vi "PC-Beamage Labview Example.vi"() -> ()   [LabVIEW 2013]
panel:
  in  "Manual":bool
  in  "Auto":bool
  in  "save current image":bool caption="Capture"
  in  "subtract background":bool caption="Capture"
  in  "ms":dbl=200.0 min=0.06 max=200.0 step=0.01
  in  "1ovre on":bool
  in  "FWHM On":bool
  in  "Log on":bool
  in  "Gauss on":bool
  in  "1ovre":bool
  in  "FWHM":bool
  in  "Log":bool
  in  "Gauss":bool caption="Press to Activate Measurements"
  in  "Display":T1(ring) caption="Press Buttons to Activate XY Measurements"
  in  "Time out":i32
  out "ok for com":bool
  out "DLL Present":bool
  out "Connected":bool
  in  "Common Measurements":T2(ring)
  out "Common Measurement":string caption="Effective Diameter"
  in  "Y Axis Measurements":T3(ring)
  in  "X Axis Measurements":T3(ring)
  out "Camera Serial Number":string
  out "PC Beamage Version":string caption="PC Beamage SW Version"
  out "Y Axis Measurement":string caption="Y Axis Centroid"
  out "X Axis Measurement":string caption="X Axis Centroid"
  in  "exit":bool
  in  "Orientation :":enum16{"Auto Orient", "0 Degrees", "45 Degress"}(ring)
  in  "Center :":enum16{"Centroid", "Peak"}(ring)
  in  "start capture":bool caption="Capture"
  in  "disconnect":bool
  in  "connect":bool
  in  "Definition :":T4(ring)
  # "PC-Beamage Labview Control Example"
  # "Main Controls"
  # "Measures"
  # "Exposure Time"
  # "Select Measurements to Display"
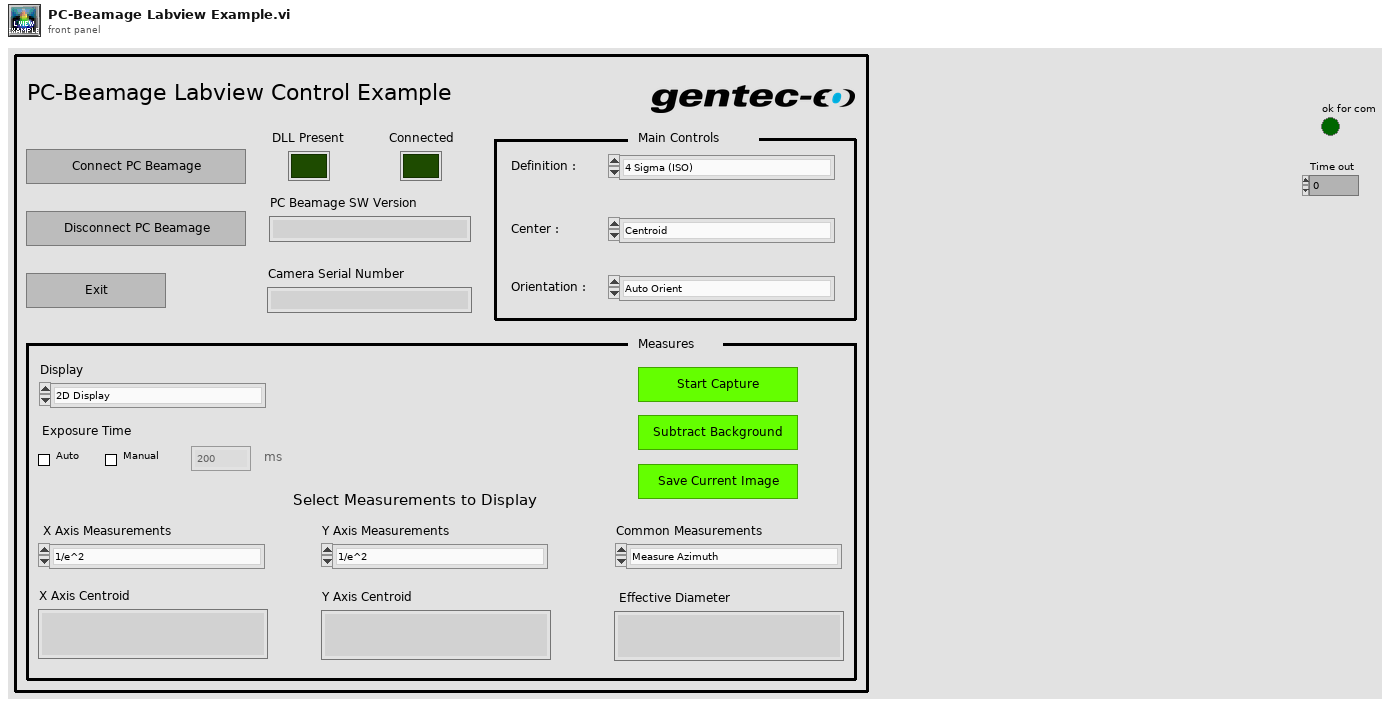
[diagram p1: front panel]
types:
  T1 = enum16{"2D Display", "3D Display", "XY Display", "Beam Track Display"}
  T2 = enum16{"Measure Azimuth", "Measure Delta", "Measure Effective Diameter", "Measure Ellipticity", "Measure Number of Samples", "Measure Orientation", "Measure Peak Saturation", "Measure Minor Axis", "Measure Major Axis", "Measure RMS", ""}
  T3 = enum16{"1/e^2", "Centroid", "Delta", "FWHM", "Gaussian Equation", "Gaussian % Fit", "Roughness Fit", "Last", "Mean", "Peak to Average Ratio", "Peak"}
  T4 = enum16{"4 Sigma (ISO)", "FWHM along Crosshairs (50%)", "1 / e^2 along Crosshairs (13.5%)", "86 % effective Diameter"}
  T5 = enum8{"Enabled", "Disabled", "Disabled and Grayed Out"}
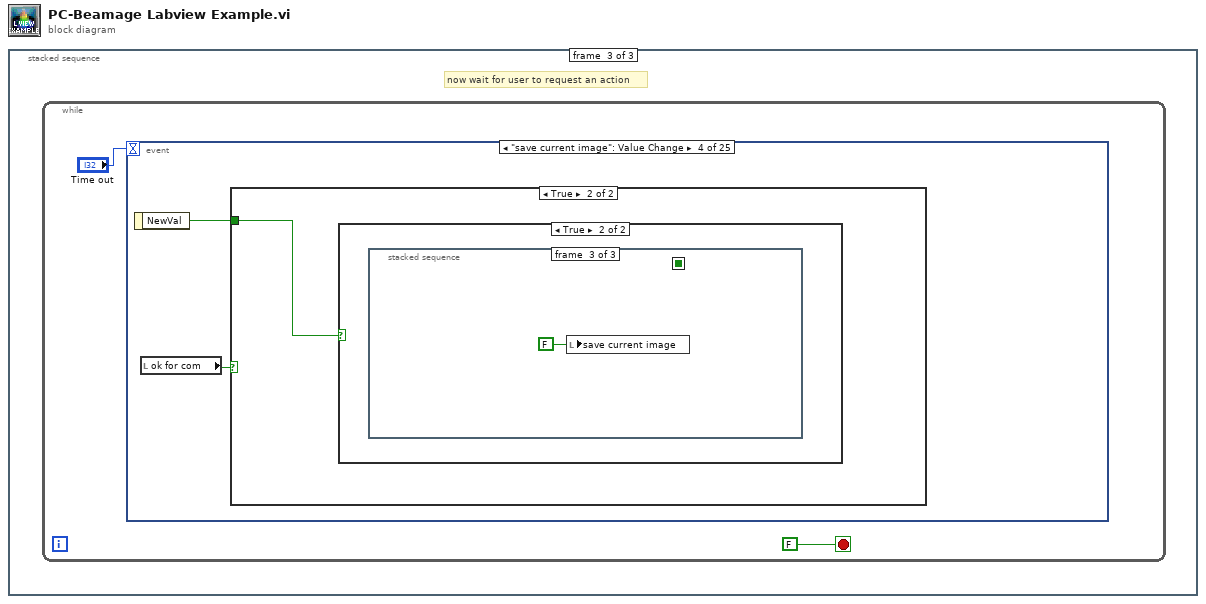
[diagram p0: block diagram]
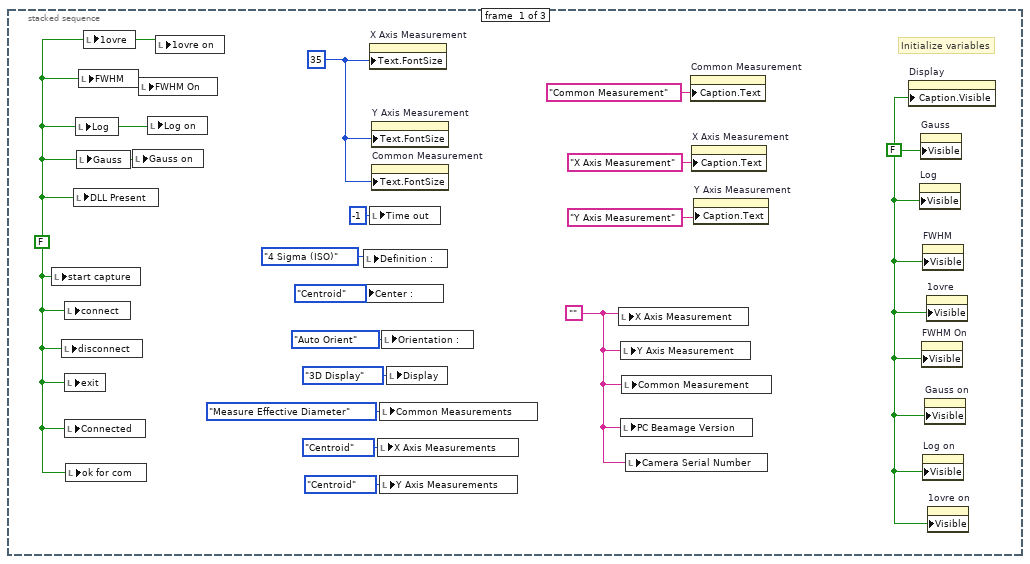
[diagram p2: hidden frame]
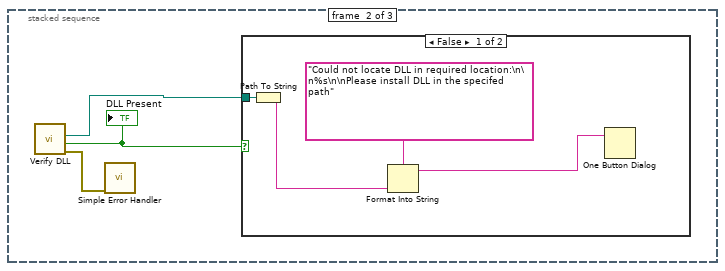
[diagram p3: hidden frame]
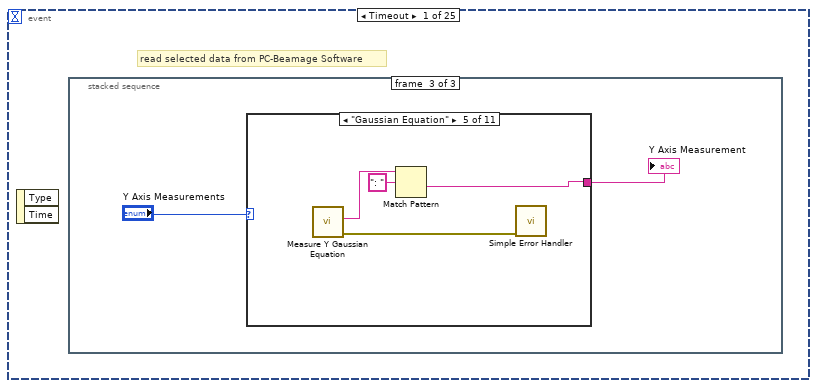
[diagram p5: hidden frame]
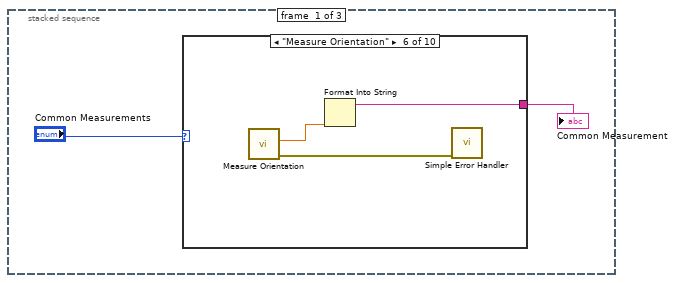
[diagram p6: hidden frame]
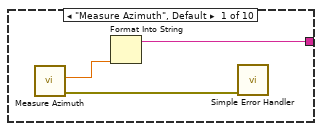
[diagram p7: hidden frame]
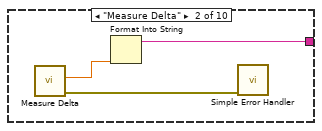
[diagram p8: hidden frame]
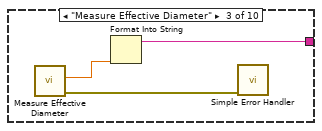
[diagram p9: hidden frame]
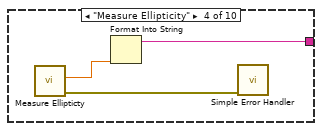
[diagram p10: hidden frame]
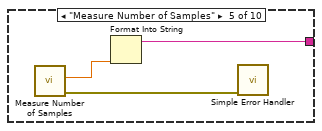
[diagram p11: hidden frame]
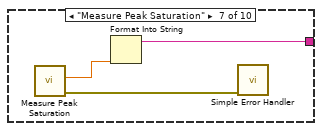
[diagram p12: hidden frame]
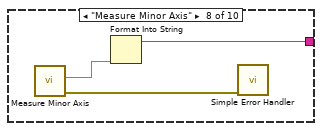
[diagram p13: hidden frame]
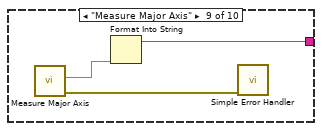
[diagram p14: hidden frame]
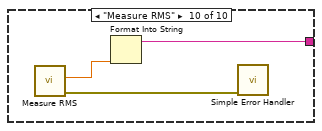
[diagram p15: hidden frame]
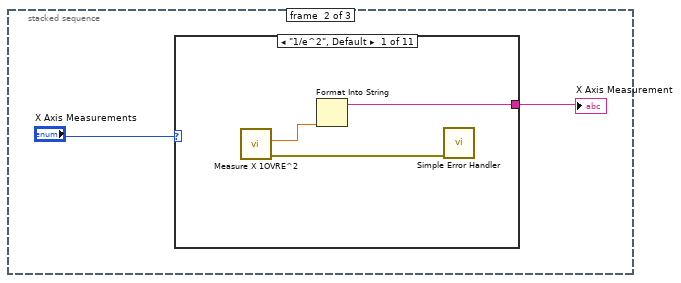
[diagram p16: hidden frame]
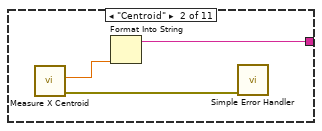
[diagram p17: hidden frame]
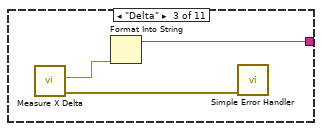
[diagram p18: hidden frame]
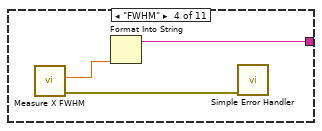
[diagram p19: hidden frame]
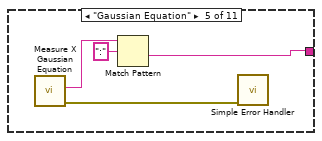
[diagram p20: hidden frame]
diagram:
  n1 = stacked-sequence {
    frame #0 {
      w3 = FALSE ("Visible")
      w7 = u32 35 ("Text.Font:Size")
      w4 = FALSE ("verifiy dll")
      w15 = ""
      # "Initialize variables"
      n2 = local write "start capture"(w4) -> ()
      n3 = local write "disconnect"(w4) -> ()
      n4 = local write "connect"(w4) -> ()
      n5 = local write "exit"(w4) -> ()
      n6 = local write "Connected"(w4) -> ()
      n7 = local write "ok for com"(w4) -> ()
      n8 = local write "DLL Present"(w4) -> ()
      n9 = local write "Log"(w4) -> ()
      n10 = local write "Gauss"(w4) -> ()
      n11 = local write "FWHM"(w4) -> ()
      n12 = local write "1ovre"(w4) -> ()
      n13 = local write "Gauss on"(w4) -> ()
      n14 = local write "FWHM On"(w4) -> ()
      n15 = local write "Log on"(w4) -> ()
      n16 = local write "1ovre on"(w4) -> ()
      n17 = local write "Center :"(enum16{"Centroid", "Peak"}."Centroid" ("Center :")) -> ()
      n18 = local write "Definition :"(T4."4 Sigma (ISO)" ("Definition :")) -> ()
      n19 = property on="X Axis Measurement" class="Str"("Text.FontSize"=w7) -> ()  [unwired: 2 in, 2 out]
      n20 = local write "Time out"(-1 ("Time out")) -> ()
      n21 = property on="Y Axis Measurement" class="Str"("Text.FontSize"=w7) -> ()  [unwired: 2 in, 2 out]
      n22 = property on="Common Measurement" class="Str"("Text.FontSize"=w7) -> ()  [unwired: 2 in, 2 out]
      n23 = local write "X Axis Measurements"(T3."Centroid" ("X Axis Measurements")) -> ()
      n24 = local write "Common Measurements"(T2."Measure Effective Diameter" ("Common Measurements")) -> ()
      n25 = local write "Y Axis Measurements"(T3."Centroid" ("Y Axis Measurements")) -> ()
      n26 = local write "Orientation :"(enum16{"Auto Orient", "0 Degrees", "45 Degress"}."Auto Orient" ("Orientation :")) -> ()
      n27 = local write "Display"(T1."3D Display" ("Display")) -> ()
      n28 = local write "X Axis Measurement"(w15) -> ()
      n29 = local write "Y Axis Measurement"(w15) -> ()
      n30 = local write "PC Beamage Version"(w15) -> ()
      n31 = local write "Common Measurement"(w15) -> ()
      n32 = local write "Camera Serial Number"(w15) -> ()
      n33 = property on="Common Measurement" class="Str"("Caption.Text"="Common Measurement") -> ()  [unwired: 2 in, 2 out]
      n34 = property on="X Axis Measurement" class="Str"("Caption.Text"="X Axis Measurement") -> ()  [unwired: 2 in, 2 out]
      n35 = property on="Y Axis Measurement" class="Str"("Caption.Text"="Y Axis Measurement") -> ()  [unwired: 2 in, 2 out]
      n36 = property on="Display" class="Enum (strict)"("Caption.Visible"=w3) -> ()  [unwired: 2 in, 2 out]
      n37 = property on="Log" class="Bool (strict)"("Visible"=w3) -> ()  [unwired: 2 in, 2 out]
      n38 = property on="Gauss" class="Bool (strict)"("Visible"=w3) -> ()  [unwired: 2 in, 2 out]
      n39 = property on="FWHM On" class="Bool (strict)"("Visible"=w3) -> ()  [unwired: 2 in, 2 out]
      n40 = property on="FWHM" class="Bool (strict)"("Visible"=w3) -> ()  [unwired: 2 in, 2 out]
      n41 = property on="Log on" class="Bool (strict)"("Visible"=w3) -> ()  [unwired: 2 in, 2 out]
      n42 = property on="Gauss on" class="Bool (strict)"("Visible"=w3) -> ()  [unwired: 2 in, 2 out]
      n43 = property on="1ovre" class="Bool (strict)"("Visible"=w3) -> ()  [unwired: 2 in, 2 out]
      n44 = property on="1ovre on" class="Bool (strict)"("Visible"=w3) -> ()  [unwired: 2 in, 2 out]
    }
    frame #1 {
      n45 = call "Verify DLL.vi"() -> ("error out"=w16:errorcluster, "DLL is Present"=w18:bool, "path"=w17:path)  [unwired: 9 in]
      "DLL Present" <- w18
      n46 = call <vilib>:"Simple Error Handler.vi"("error in (no error)"=w16) -> ()  [unwired: 4 in, 5 out]
      n47 = case shown="False" w18 {
        tunnel: w17 -> [w22 _]
        frame False {
          n48 = Path To String(path=w22) -> (string=w20:string)
          n49 = Format Into String(format string="Could not locate DLL in required location:\n\n%s\n\nPlease install DLL in the specifed path", w20) -> (resulting string=w19:string)  [unwired: 2 in, 1 out]
          n50 = One Button Dialog(message=w19) -> ()  [unwired: 1 in, 1 out]
        }
        frame True {
        }
      }
    }
    frame #2 {
      # "now wait for user to request an action"
      n51 = while {
        stop <- FALSE stop-if-true
        n52 = event shown="[3] \"save current image\": Value Change" {
          selector: _ -> [_ _ _ _ _ _ _ _ _ _ _ _ _ _ _ _ _ _ _ _ _ _ _ _ _]
          dyn-events: _ -> [_ _ _ _ _ _ _ _ _ _ _ _ _ _ _ _ _ _ _ _ _ _ _ _ _]
          timeout: "Time out" -> [_ _ _ _ _ _ _ _ _ _ _ _ _ _ _ _ _ _ _ _ _ _ _ _ _]
          event Timeout {
            # "read selected data from PC-Beamage Software"
            n53 = event-data() -> ()  [unwired: 1 in, 2 out]
            n54 = stacked-sequence {
              frame #0 {
                n55 = case shown="\"Measure Orientation\"" "Common Measurements" {
                  tunnel: [w27 w30 w33 w36 w39 w42 w45 w48 w51 w54] -> w25
                  frame "Measure Azimuth", Default {
                    n56 = call "Measure Azimuth.vi"() -> ("error out"=w29:errorcluster, "Azimuth"=w28:dbl)  [unwired: 10 in]
                    n57 = Format Into String(w28) -> (resulting string=w27:string)  [unwired: 3 in, 1 out]
                    n58 = call <vilib>:"Simple Error Handler.vi"("error in (no error)"=w29) -> ()  [unwired: 4 in, 5 out]
                  }
                  frame "Measure Delta" {
                    n59 = call "Measure Delta.vi"() -> ("error out"=w32:errorcluster, "Delta"=w31:dbl)  [unwired: 10 in]
                    n60 = Format Into String(w31) -> (resulting string=w30:string)  [unwired: 3 in, 1 out]
                    n61 = call <vilib>:"Simple Error Handler.vi"("error in (no error)"=w32) -> ()  [unwired: 4 in, 5 out]
                  }
                  frame "Measure Effective Diameter" {
                    n62 = call "Measure Effective Diameter.vi"() -> ("error out"=w35:errorcluster, "Effective Diameter"=w34:dbl)  [unwired: 10 in]
                    n63 = Format Into String(w34) -> (resulting string=w33:string)  [unwired: 3 in, 1 out]
                    n64 = call <vilib>:"Simple Error Handler.vi"("error in (no error)"=w35) -> ()  [unwired: 4 in, 5 out]
                  }
                  frame "Measure Ellipticity" {
                    n65 = call "Measure Ellipticty.vi"() -> ("error out"=w38:errorcluster, "Ellipticity"=w37:dbl)  [unwired: 10 in]
                    n66 = Format Into String(w37) -> (resulting string=w36:string)  [unwired: 3 in, 1 out]
                    n67 = call <vilib>:"Simple Error Handler.vi"("error in (no error)"=w38) -> ()  [unwired: 4 in, 5 out]
                  }
                  frame "Measure Number of Samples" {
                    n68 = call "Measure Number of Samples.vi"() -> ("error out"=w41:errorcluster, "Number of Samples"=w40:dbl)  [unwired: 10 in]
                    n69 = Format Into String(w40) -> (resulting string=w39:string)  [unwired: 3 in, 1 out]
                    n70 = call <vilib>:"Simple Error Handler.vi"("error in (no error)"=w41) -> ()  [unwired: 4 in, 5 out]
                  }
                  frame "Measure Orientation" {
                    n71 = call "Measure Orientation.vi"() -> ("error out"=w44:errorcluster, "Orienttion"=w43:dbl)  [unwired: 10 in]
                    n72 = Format Into String(w43) -> (resulting string=w42:string)  [unwired: 3 in, 1 out]
                    n73 = call <vilib>:"Simple Error Handler.vi"("error in (no error)"=w44) -> ()  [unwired: 4 in, 5 out]
                  }
                  frame "Measure Peak Saturation" {
                    n74 = call "Measure Peak Saturation.vi"() -> ("error out"=w47:errorcluster, "Peak Saturation"=w46:dbl)  [unwired: 10 in]
                    n75 = Format Into String(w46) -> (resulting string=w45:string)  [unwired: 3 in, 1 out]
                    n76 = call <vilib>:"Simple Error Handler.vi"("error in (no error)"=w47) -> ()  [unwired: 4 in, 5 out]
                  }
                  frame "Measure Minor Axis" {
                    n77 = call "Measure Minor Axis.vi"() -> ("error out"=w50:errorcluster, "Minor Axis"=w49:dbl)  [unwired: 10 in]
                    n78 = Format Into String(w49) -> (resulting string=w48:string)  [unwired: 3 in, 1 out]
                    n79 = call <vilib>:"Simple Error Handler.vi"("error in (no error)"=w50) -> ()  [unwired: 4 in, 5 out]
                  }
                  frame "Measure Major Axis" {
                    n80 = call "Measure Major Axis.vi"() -> ("error out"=w53:errorcluster, "Major Axis"=w52:dbl)  [unwired: 10 in]
                    n81 = Format Into String(w52) -> (resulting string=w51:string)  [unwired: 3 in, 1 out]
                    n82 = call <vilib>:"Simple Error Handler.vi"("error in (no error)"=w53) -> ()  [unwired: 4 in, 5 out]
                  }
                  frame "Measure RMS" {
                    n83 = call "Measure RMS.vi"() -> ("error out"=w56:errorcluster, "RMS"=w55:dbl)  [unwired: 10 in]
                    n84 = Format Into String(w55) -> (resulting string=w54:string)  [unwired: 3 in, 1 out]
                    n85 = call <vilib>:"Simple Error Handler.vi"("error in (no error)"=w56) -> ()  [unwired: 4 in, 5 out]
                  }
                }
                "Common Measurement" <- w25
              }
              frame #1 {
                n86 = case shown="\"1/e^2\", Default" "X Axis Measurements" {
                  tunnel: [w59 w62 w65 w68 w71 w75 w78 w81 w84 w87 w90] -> w58
                  frame "1/e^2", Default {
                    n87 = call "Measure X 1OVRE^2.vi"() -> ("error out"=w61:errorcluster, "X 1/E^2"=w60:dbl)  [unwired: 10 in]
                    n88 = Format Into String(w60) -> (resulting string=w59:string)  [unwired: 3 in, 1 out]
                    n89 = call <vilib>:"Simple Error Handler.vi"("error in (no error)"=w61) -> ()  [unwired: 4 in, 5 out]
                  }
                  frame "Centroid" {
                    n90 = call "Measure X Centroid.vi"() -> ("error out"=w64:errorcluster, "X Centroid"=w63:dbl)  [unwired: 10 in]
                    n91 = Format Into String(w63) -> (resulting string=w62:string)  [unwired: 3 in, 1 out]
                    n92 = call <vilib>:"Simple Error Handler.vi"("error in (no error)"=w64) -> ()  [unwired: 4 in, 5 out]
                  }
                  frame "Delta" {
                    n93 = call "Measure X Delta.vi"() -> ("error out"=w67:errorcluster, "X Delta"=w66:dbl)  [unwired: 10 in]
                    n94 = Format Into String(w66) -> (resulting string=w65:string)  [unwired: 3 in, 1 out]
                    n95 = call <vilib>:"Simple Error Handler.vi"("error in (no error)"=w67) -> ()  [unwired: 4 in, 5 out]
                  }
                  frame "FWHM" {
                    n96 = call "Measure X FWHM.vi"() -> ("error out"=w70:errorcluster, "X FWHM"=w69:dbl)  [unwired: 10 in]
                    n97 = Format Into String(w69) -> (resulting string=w68:string)  [unwired: 3 in, 1 out]
                    n98 = call <vilib>:"Simple Error Handler.vi"("error in (no error)"=w70) -> ()  [unwired: 4 in, 5 out]
                  }
                  frame "Gaussian Equation" {
                    n99 = call "Measure X Gaussian Equation.vi"() -> ("error out"=w74:errorcluster, "X Gaussian Equation"=w73:string)  [unwired: 10 in]
                    n100 = Match Pattern(string=w73, regular expression=":") -> (after substring=w71:string)  [unwired: 1 in, 3 out]
                    n101 = call <vilib>:"Simple Error Handler.vi"("error in (no error)"=w74) -> ()  [unwired: 4 in, 5 out]
                  }
                  frame "Gaussian % Fit" {
                    n102 = call "Measure X Gaussian Fit %.vi"() -> ("error out"=w77:errorcluster, "X Gaussian Fit %"=w76:dbl)  [unwired: 10 in]
                    n103 = Format Into String(w76) -> (resulting string=w75:string)  [unwired: 3 in, 1 out]
                    n104 = call <vilib>:"Simple Error Handler.vi"("error in (no error)"=w77) -> ()  [unwired: 4 in, 5 out]
                  }
                  frame "Roughness Fit" {
                    n105 = call "Measure X Roughness Fit.vi"() -> ("error out"=w80:errorcluster, "X Roughness Fit"=w79:dbl)  [unwired: 10 in]
                    n106 = Format Into String(w79) -> (resulting string=w78:string)  [unwired: 3 in, 1 out]
                    n107 = call <vilib>:"Simple Error Handler.vi"("error in (no error)"=w80) -> ()  [unwired: 4 in, 5 out]
                  }
                  frame "Last" {
                    n108 = call "Measure X Last.vi"() -> ("error out"=w83:errorcluster, "X Last"=w82:dbl)  [unwired: 10 in]
                    n109 = Format Into String(w82) -> (resulting string=w81:string)  [unwired: 3 in, 1 out]
                    n110 = call <vilib>:"Simple Error Handler.vi"("error in (no error)"=w83) -> ()  [unwired: 4 in, 5 out]
                  }
                  frame "Mean" {
                    n111 = call "Measure X Mean.vi"() -> ("error out"=w86:errorcluster, "X Mean"=w85:dbl)  [unwired: 10 in]
                    n112 = Format Into String(w85) -> (resulting string=w84:string)  [unwired: 3 in, 1 out]
                    n113 = call <vilib>:"Simple Error Handler.vi"("error in (no error)"=w86) -> ()  [unwired: 4 in, 5 out]
                  }
                  frame "Peak to Average Ratio" {
                    n114 = call "Measure X Peak to Average.vi"() -> ("error out"=w89:errorcluster, "X Peak to Average Ratio"=w88:dbl)  [unwired: 10 in]
                    n115 = Format Into String(w88) -> (resulting string=w87:string)  [unwired: 3 in, 1 out]
                    n116 = call <vilib>:"Simple Error Handler.vi"("error in (no error)"=w89) -> ()  [unwired: 4 in, 5 out]
                  }
                  frame "Peak" {
                    n117 = call "Measure X Peak.vi"() -> ("error out"=w92:errorcluster, "X Peak"=w91:dbl)  [unwired: 10 in]
                    n118 = Format Into String(w91) -> (resulting string=w90:string)  [unwired: 3 in, 1 out]
                    n119 = call <vilib>:"Simple Error Handler.vi"("error in (no error)"=w92) -> ()  [unwired: 4 in, 5 out]
                  }
                }
                "X Axis Measurement" <- w58
              }
              frame #2 {
                n120 = case shown="\"Gaussian Equation\"" "Y Axis Measurements" {
                  tunnel: [w95 w98 w101 w104 w107 w111 w114 w117 w120 w123 w126] -> w93
                  frame "1/e^2", Default {
                    n121 = call "Measure Y 1OVRE^2.vi"() -> ("error out"=w97:errorcluster, "Y 1/E^2"=w96:dbl)  [unwired: 10 in]
                    n122 = Format Into String(w96) -> (resulting string=w95:string)  [unwired: 3 in, 1 out]
                    n123 = call <vilib>:"Simple Error Handler.vi"("error in (no error)"=w97) -> ()  [unwired: 4 in, 5 out]
                  }
                  frame "Centroid" {
                    n124 = call "Measure Y Centroid.vi"() -> ("error out"=w100:errorcluster, "Y Centroid"=w99:dbl)  [unwired: 10 in]
                    n125 = Format Into String(w99) -> (resulting string=w98:string)  [unwired: 3 in, 1 out]
                    n126 = call <vilib>:"Simple Error Handler.vi"("error in (no error)"=w100) -> ()  [unwired: 4 in, 5 out]
                  }
                  frame "Delta" {
                    n127 = call "Measure Y Delta.vi"() -> ("error out"=w103:errorcluster, "Y Delta"=w102:dbl)  [unwired: 10 in]
                    n128 = Format Into String(w102) -> (resulting string=w101:string)  [unwired: 3 in, 1 out]
                    n129 = call <vilib>:"Simple Error Handler.vi"("error in (no error)"=w103) -> ()  [unwired: 4 in, 5 out]
                  }
                  frame "FWHM" {
                    n130 = call "Measure Y FWHM.vi"() -> ("error out"=w106:errorcluster, "Y FWHM"=w105:dbl)  [unwired: 10 in]
                    n131 = Format Into String(w105) -> (resulting string=w104:string)  [unwired: 3 in, 1 out]
                    n132 = call <vilib>:"Simple Error Handler.vi"("error in (no error)"=w106) -> ()  [unwired: 4 in, 5 out]
                  }
                  frame "Gaussian Equation" {
                    n133 = call "Measure Y Gaussian Equation.vi"() -> ("error out"=w110:errorcluster, "Y Gaussian Equation"=w109:string)  [unwired: 10 in]
                    n134 = Match Pattern(string=w109, regular expression=": ") -> (after substring=w107:string)  [unwired: 1 in, 3 out]
                    n135 = call <vilib>:"Simple Error Handler.vi"("error in (no error)"=w110) -> ()  [unwired: 4 in, 5 out]
                  }
                  frame "Gaussian % Fit" {
                    n136 = call "Measure Y Gaussian Fit %.vi"() -> ("error out"=w113:errorcluster, "Y Gaussian Fit %"=w112:dbl)  [unwired: 10 in]
                    n137 = Format Into String(w112) -> (resulting string=w111:string)  [unwired: 3 in, 1 out]
                    n138 = call <vilib>:"Simple Error Handler.vi"("error in (no error)"=w113) -> ()  [unwired: 4 in, 5 out]
                  }
                  frame "Roughness Fit" {
                    n139 = call "Measure Y Roughness Fit.vi"() -> ("error out"=w116:errorcluster, "Y Roughness Fit"=w115:dbl)  [unwired: 10 in]
                    n140 = Format Into String(w115) -> (resulting string=w114:string)  [unwired: 3 in, 1 out]
                    n141 = call <vilib>:"Simple Error Handler.vi"("error in (no error)"=w116) -> ()  [unwired: 4 in, 5 out]
                  }
                  frame "Last" {
                    n142 = call "Measure Y Last.vi"() -> ("error out"=w119:errorcluster, "Y Last"=w118:dbl)  [unwired: 10 in]
                    n143 = Format Into String(w118) -> (resulting string=w117:string)  [unwired: 3 in, 1 out]
                    n144 = call <vilib>:"Simple Error Handler.vi"("error in (no error)"=w119) -> ()  [unwired: 4 in, 5 out]
                  }
                  frame "Mean" {
                    n145 = call "Measure Y Mean.vi"() -> ("error out"=w122:errorcluster, "Y Mean"=w121:dbl)  [unwired: 10 in]
                    n146 = Format Into String(w121) -> (resulting string=w120:string)  [unwired: 3 in, 1 out]
                    n147 = call <vilib>:"Simple Error Handler.vi"("error in (no error)"=w122) -> ()  [unwired: 4 in, 5 out]
                  }
                  frame "Peak to Average Ratio" {
                    n148 = call "Measure Y Peak to Average.vi"() -> ("error out"=w125:errorcluster, "Y Peak to Average Ratio"=w124:dbl)  [unwired: 10 in]
                    n149 = Format Into String(w124) -> (resulting string=w123:string)  [unwired: 3 in, 1 out]
                    n150 = call <vilib>:"Simple Error Handler.vi"("error in (no error)"=w125) -> ()  [unwired: 4 in, 5 out]
                  }
                  frame "Peak" {
                    n151 = call "Measure Y Peak.vi"() -> ("error out"=w128:errorcluster, "Y Peak"=w127:dbl)  [unwired: 10 in]
                    n152 = Format Into String(w127) -> (resulting string=w126:string)  [unwired: 3 in, 1 out]
                    n153 = call <vilib>:"Simple Error Handler.vi"("error in (no error)"=w128) -> ()  [unwired: 4 in, 5 out]
                  }
                }
                "Y Axis Measurement" <- w93
              }
            }
          }
          event "connect": Value Change {
            n154 = event-data() -> ()  [unwired: 1 in, 1 out]
            n155 = stacked-sequence {
              frame #0 {
                n156 = call "Connect to PC Beamage.vi"() -> ("error out"=w130:errorcluster, "Connected"=w131:bool)  [unwired: 10 in]
                "Connected" <- w131
                n157 = case shown="True" w131 {
                  tunnel: w130 -> [w133 w135]
                  tunnel: [w133 w138] -> w129
                  frame False {
                    n158 = One Button Dialog(message="Connection Failed. Verify PC Beamage 3.0 is\nrunning and the Labview Pipe is Open.\n\nShow/Hide\n  Options\n>Start Labview Pipeline") -> ()  [unwired: 1 in, 1 out]
                  }
                  frame True {
                    n159 = call "Control Stop Capture.vi"("error in"=w135) -> ("error out"=w134:errorcluster)  [unwired: 8 in, 2 out]
                    n160 = call "Query PC Beamage Version.vi"("error in"=w134) -> ("error out"=w139:errorcluster, "PC Beamage Version"=→"PC Beamage Version":string)  [unwired: 9 in]
                    n161 = call "Query Serial Number.vi"("error in"=w139) -> ("error out"=w138:errorcluster, "Serial Number"=→"Camera Serial Number":string)  [unwired: 9 in]
                  }
                }
                n162 = call <vilib>:"Simple Error Handler.vi"("error in (no error)"=w129) -> ()  [unwired: 4 in, 5 out]
              }
              frame #1 {
                w140 = FALSE ("verifiy dll")
                n163 = local read "Connected"() -> (w142:bool)
                n164 = local read "DLL Present"() -> (w143:bool)
                n165 = local write "connect"(w140) -> ()
                n166 = local write "start capture"(w140) -> ()
                n167 = And(x=w143, y=w142) -> (x .and. y?=→"ok for com":bool)
              }
              frame #2 {
                # "put PC-Beamage sync with labview"
                n168 = local read "ok for com"() -> (w144:bool)
                n169 = case shown="True" w144 {
                  frame False {
                  }
                  frame True {
                    w148 = FALSE ("Manual")
                    n170 = local write "Manual"(w148) -> ()
                    n171 = local write "Center :"(enum16{"Centroid", "Peak"}."Centroid" ("Center :")) -> ()
                    n172 = local write "X Axis Measurements"(T3."Centroid" ("X Axis Measurements")) -> ()
                    n173 = local write "subtract background"(w148) -> ()
                    n174 = local write "Orientation :"(enum16{"Auto Orient", "0 Degrees", "45 Degress"}."Auto Orient" ("Orientation :")) -> ()
                    n175 = local write "save current image"(w148) -> ()
                    n176 = local write "Common Measurements"(T2."Measure Effective Diameter" ("Common Measurements")) -> ()
                    n177 = local write "Y Axis Measurements"(T3."Centroid" ("Y Axis Measurements")) -> ()
                    n178 = local write "Display"(T1."3D Display" ("Display")) -> ()
                    n179 = local write "Definition :"(T4."4 Sigma (ISO)" ("Definition :")) -> ()
                    n180 = local write "Auto"(TRUE ("Auto")) -> ()
                    n181 = property on="save current image" class="Bool (strict)"("DisabledEnum"=T5."Enabled" ("Disabled")) -> ()  [unwired: 2 in, 2 out]
                    n182 = local write "ms"(50.0 ("ms")) -> ()
                    n183 = property on="ms" class="DigNum (strict)"("DisabledEnum"=T5."Disabled and Grayed Out" ("Disabled")) -> ()  [unwired: 2 in, 2 out]
                  }
                }
              }
              frame #3 {
                # "put PC-Beamage sync with labview"
                n184 = local read "ok for com"() -> (w157:bool)
                n185 = case shown="True" w157 {
                  frame False {
                  }
                  frame True {
                    n186 = property on="Common Measurements" class="Enum (strict)"() -> ("RingText.Text"=w160:string)  [unwired: 2 in, 2 out]
                    n187 = Match Pattern(string=w160, regular expression="Measure") -> (after substring=w158:string)  [unwired: 1 in, 3 out]
                    n188 = property on="Common Measurement" class="Str"("Caption.Text"=w158) -> ()  [unwired: 2 in, 2 out]
                  }
                }
              }
              frame #4 {
                # "put PC-Beamage sync with labview"
                n189 = local read "ok for com"() -> (w161:bool)
                n190 = case shown="True" w161 {
                  frame False {
                  }
                  frame True {
                    n191 = property on="X Axis Measurements" class="Enum (strict)"() -> ("RingText.Text"=w164:string)  [unwired: 2 in, 2 out]
                    n192 = Format Into String(format string="X Axis %s", w164) -> (resulting string=w162:string)  [unwired: 2 in, 1 out]
                    n193 = property on="X Axis Measurement" class="Str"("Caption.Text"=w162) -> ()  [unwired: 2 in, 2 out]
                  }
                }
              }
              frame #5 {
                # "put PC-Beamage sync with labview"
                n194 = local read "ok for com"() -> (w165:bool)
                n195 = case shown="True" w165 {
                  frame False {
                  }
                  frame True {
                    n196 = property on="Y Axis Measurements" class="Enum (strict)"() -> ("RingText.Text"=w168:string)  [unwired: 2 in, 2 out]
                    n197 = Format Into String(format string="Y Axis %s", w168) -> (resulting string=w166:string)  [unwired: 2 in, 1 out]
                    n198 = property on="Y Axis Measurement" class="Str"("Caption.Text"=w166) -> ()  [unwired: 2 in, 2 out]
                  }
                }
              }
              frame #6 {
                # "put PC-Beamage sync with labview"
                n199 = local read "ok for com"() -> (w169:bool)
                n200 = case shown="True" w169 {
                  frame False {
                  }
                  frame True {
                    n201 = call "Control 4 Sigma.vi"() -> ("error out"=w175:errorcluster)  [unwired: 9 in, 2 out]
                    n202 = call "Control Centroid.vi"("error in"=w175) -> ("error out"=w176:errorcluster)  [unwired: 8 in, 2 out]
                    n203 = call "Control Auto.vi"("error in"=w176) -> ("error out"=w174:errorcluster)  [unwired: 8 in, 2 out]
                    n204 = call "Display 3D.vi"("error in"=w174) -> ("error out"=w173:errorcluster)  [unwired: 8 in, 2 out]
                    n205 = call "Activate LIN.vi"("error in"=w173) -> ("error out"=w170:errorcluster)  [unwired: 8 in, 2 out]
                    n206 = call "Control Auto Exposure.vi"("error in"=w170) -> ("error out"=w172:errorcluster)  [unwired: 8 in, 2 out]
                    n207 = local read "ms"() -> (w171:dbl)
                    n208 = call "Send Exposure Time.vi"("error in"=w172, "Exposure Time (ms)"=w171) -> ()  [unwired: 7 in, 3 out]
                  }
                }
              }
            }
          }
          event "start capture": Value Change {
            n209 = event-data() -> ("NewVal"=w177:bool)  [unwired: 1 in]
            n210 = local read "ok for com"() -> (w178:bool)
            n211 = case shown="True" w178 {
              tunnel: w177 -> [_ w181]
              frame False {
                n212 = local write "Time out"(-1 ("Time out")) -> ()
                n213 = One Button Dialog(message="Not connected to PC-Beamage Software") -> ()  [unwired: 1 in, 1 out]
              }
              frame True {
                n214 = case shown="True" w181 {
                  frame False {
                    n215 = stacked-sequence {
                      frame #0 {
                        n216 = call "Control Stop Capture.vi"() -> ("error out"=w182:errorcluster)  [unwired: 9 in, 2 out]
                        n217 = local write "Time out"(-1 ("Time out")) -> ()
                        n218 = call <vilib>:"Simple Error Handler.vi"("error in (no error)"=w182) -> ()  [unwired: 4 in, 5 out]
                      }
                      frame #1 {
                        n219 = property on="save current image" class="Bool (strict)"("DisabledEnum"=T5."Enabled" ("Disabled")) -> ()  [unwired: 2 in, 2 out]
                      }
                    }
                  }
                  frame True {
                    n220 = stacked-sequence {
                      frame #0 {
                        # "every 333ms we will go to time out event and get selected data"
                        n221 = call "Control Start Capture.vi"() -> ("error out"=w185:errorcluster)  [unwired: 9 in, 2 out]
                        n222 = local write "Time out"(333 ("Time out")) -> ()
                        n223 = call <vilib>:"Simple Error Handler.vi"("error in (no error)"=w185) -> ()  [unwired: 4 in, 5 out]
                      }
                      frame #1 {
                        n224 = property on="save current image" class="Bool (strict)"("DisabledEnum"=T5."Disabled and Grayed Out" ("Disabled")) -> ()  [unwired: 2 in, 2 out]
                      }
                    }
                  }
                }
              }
            }
          }
          event "save current image": Value Change {
            n225 = event-data() -> ("NewVal"=w188:bool)  [unwired: 1 in]
            n226 = local read "ok for com"() -> (w189:bool)
            n227 = case shown="True" w189 {
              tunnel: w188 -> [_ w192]
              frame False {
                n228 = local write "Time out"(-1 ("Time out")) -> ()
                n229 = One Button Dialog(message="Not connected to PC-Beamage Software") -> ()  [unwired: 1 in, 1 out]
              }
              frame True {
                n230 = case shown="True" w192 {
                  frame False {
                  }
                  frame True {
                    n231 = stacked-sequence {
                      seq-local: [w193 _ _] -> [_ w194 _]
                      frame #0 {
                        n232 = call "File Format Selection"() -> ("Save as Bitmap"=w193:bool)  [unwired: 18 in, 1 out]
                      }
                      frame #1 {
                        n233 = case shown="False" w194 {
                          tunnel: [w196 w197] -> w195
                          frame False {
                            n234 = call "Control Save Text.vi"() -> ("error out"=w196:errorcluster)  [unwired: 9 in, 2 out]
                          }
                          frame True {
                            n235 = call "Control Save Image.vi"() -> ("error out"=w197:errorcluster)  [unwired: 9 in, 2 out]
                          }
                        }
                        n236 = call <vilib>:"Simple Error Handler.vi"("error in (no error)"=w195) -> ()  [unwired: 4 in, 5 out]
                      }
                      frame #2 {
                        n237 = local write "save current image"(FALSE ("save current image")) -> ()
                      }
                    }
                  }
                }
              }
            }
          }
          event "Auto": Value Change {
            n238 = event-data() -> ("NewVal"=w199:bool)  [unwired: 1 in]
            n239 = local read "ok for com"() -> (w200:bool)
            n240 = case shown="False" w200 {
              tunnel: w199 -> [_ w203]
              frame False {
                n241 = local write "Time out"(-1 ("Time out")) -> ()
                n242 = One Button Dialog(message="Not connected to PC-Beamage Software") -> ()  [unwired: 1 in, 1 out]
              }
              frame True {
                n243 = case shown="True" w203 {
                  frame False {
                    # "can't unclick it, must set manual to set this to false"
                    n244 = local write "Manual"(FALSE ("Manual")) -> ()
                    n245 = local write "Auto"(TRUE ("Auto")) -> ()
                    n246 = property on="ms" class="DigNum (strict)"("DisabledEnum"=T5."Disabled and Grayed Out" ("Disabled")) -> ()  [unwired: 2 in, 2 out]
                  }
                  frame True {
                    n247 = stacked-sequence {
                      frame #0 {
                        n248 = call "Control Auto Exposure.vi"() -> ("error out"=w207:errorcluster)  [unwired: 9 in, 2 out]
                        n249 = call <vilib>:"Simple Error Handler.vi"("error in (no error)"=w207) -> ()  [unwired: 4 in, 5 out]
                      }
                      frame #1 {
                        n250 = local write "Manual"(FALSE ("Manual")) -> ()
                        n251 = property on="ms" class="DigNum (strict)"("DisabledEnum"=T5."Disabled and Grayed Out" ("Disabled")) -> ()  [unwired: 2 in, 2 out]
                      }
                    }
                  }
                }
              }
            }
          }
          event "ms": Value Change {
            n252 = event-data() -> ()  [unwired: 1 in, 1 out]
            n253 = local read "ok for com"() -> (w210:bool)
            n254 = case shown="False" w210 {
              frame False {
                n255 = local write "Time out"(-1 ("Time out")) -> ()
                n256 = One Button Dialog(message="Not connected to PC-Beamage Software") -> ()  [unwired: 1 in, 1 out]
              }
              frame True {
                n257 = call "Send Exposure Time.vi"("Exposure Time (ms)"="ms") -> ("error out"=w213:errorcluster)  [unwired: 8 in, 2 out]
                n258 = call <vilib>:"Simple Error Handler.vi"("error in (no error)"=w213) -> ()  [unwired: 4 in, 5 out]
              }
            }
          }
          event "subtract background": Value Change {
            n259 = event-data() -> ("NewVal"=w215:bool)  [unwired: 1 in]
            n260 = local read "ok for com"() -> (w216:bool)
            n261 = case shown="False" w216 {
              tunnel: w215 -> [_ w219]
              frame False {
                n262 = local write "Time out"(-1 ("Time out")) -> ()
                n263 = One Button Dialog(message="Not connected to PC-Beamage Software") -> ()  [unwired: 1 in, 1 out]
              }
              frame True {
                n264 = case shown="False" w219 {
                  frame False {
                    n265 = call "Deactivate Subtract Background.vi"() -> ("error out"=w220:errorcluster)  [unwired: 9 in, 2 out]
                    n266 = call <vilib>:"Simple Error Handler.vi"("error in (no error)"=w220) -> ()  [unwired: 4 in, 5 out]
                  }
                  frame True {
                    n267 = local read "start capture"() -> (w221:bool)
                    n268 = case shown="True" w221 {
                      frame False {
                        n269 = local write "subtract background"(FALSE ("subtract background")) -> ()
                        n270 = One Button Dialog(message="Please press Start Capture to enable the subtract background function.") -> ()  [unwired: 1 in, 1 out]
                      }
                      frame True {
                        n271 = stacked-sequence {
                          seq-local: [w224 _ _] -> [_ w226 _]
                          frame #0 {
                            n272 = Two Button Dialog(message="Please Block your laser ") -> (T button?=w224:bool)  [unwired: 2 in]
                          }
                          frame #1 {
                            n273 = case shown="True" w226 {
                              frame False {
                              }
                              frame True {
                                n274 = call "Activate Subtract Background.vi"() -> ("error out"=w227:errorcluster)  [unwired: 9 in, 2 out]
                                n275 = call <vilib>:"Simple Error Handler.vi"("error in (no error)"=w227) -> ()  [unwired: 4 in, 5 out]
                              }
                            }
                          }
                          frame #2 {
                          }
                        }
                      }
                    }
                  }
                }
              }
            }
          }
          event "Manual": Value Change {
            n276 = event-data() -> ("NewVal"=w228:bool)  [unwired: 1 in]
            n277 = local read "ok for com"() -> (w229:bool)
            n278 = case shown="False" w229 {
              tunnel: w228 -> [_ w232]
              frame False {
                n279 = local write "Time out"(-1 ("Time out")) -> ()
                n280 = One Button Dialog(message="Not connected to PC-Beamage Software") -> ()  [unwired: 1 in, 1 out]
              }
              frame True {
                n281 = case shown="True" w232 {
                  frame False {
                    # "can't unclick it, must set auto to set this to false"
                    n282 = local write "Manual"(TRUE ("Manual")) -> ()
                    n283 = local write "Auto"(FALSE ("Auto")) -> ()
                    n284 = property on="ms" class="DigNum (strict)"("DisabledEnum"=T5."Enabled" ("Disabled")) -> ()  [unwired: 2 in, 2 out]
                  }
                  frame True {
                    n285 = stacked-sequence {
                      frame #0 {
                        n286 = call "Control Manual Exposure.vi"() -> ("error out"=w237:errorcluster)  [unwired: 9 in, 2 out]
                        n287 = local read "ms"() -> (w238:dbl)
                        n288 = call "Send Exposure Time.vi"("error in"=w237, "Exposure Time (ms)"=w238) -> ("error out"=w236:errorcluster)  [unwired: 7 in, 2 out]
                        n289 = call <vilib>:"Simple Error Handler.vi"("error in (no error)"=w236) -> ()  [unwired: 4 in, 5 out]
                      }
                      frame #1 {
                        n290 = local write "Auto"(FALSE ("Manual")) -> ()
                        n291 = property on="ms" class="DigNum (strict)"("DisabledEnum"=T5."Enabled" ("Disabled")) -> ()  [unwired: 2 in, 2 out]
                      }
                    }
                  }
                }
              }
            }
          }
          event "Definition :": Value Change {
            n292 = event-data() -> ("NewVal"=w241:T4)  [unwired: 1 in]
            n293 = local read "ok for com"() -> (w242:bool)
            n294 = case shown="False" w242 {
              tunnel: w241 -> [_ w244]
              frame False {
                n295 = One Button Dialog(message="Not connected to PC-Beamage Software") -> ()  [unwired: 1 in, 1 out]
              }
              frame True {
                n296 = case shown="\"4 Sigma (ISO)\", Default" w244 {
                  frame "4 Sigma (ISO)", Default {
                    n297 = call "Control 4 Sigma.vi"() -> ("error out"=w245:errorcluster)  [unwired: 9 in, 2 out]
                    n298 = call <vilib>:"Simple Error Handler.vi"("error in (no error)"=w245) -> ()  [unwired: 4 in, 5 out]
                  }
                  frame "FWHM along Crosshairs (50%)" {
                    n299 = call "Control FWHM.vi"() -> ("error out"=w246:errorcluster)  [unwired: 9 in, 2 out]
                    n300 = call <vilib>:"Simple Error Handler.vi"("error in (no error)"=w246) -> ()  [unwired: 4 in, 5 out]
                  }
                  frame "1 / e^2 along Crosshairs (13.5%)" {
                    n301 = call "Control 1OVRe^2.vi"() -> ("error out"=w247:errorcluster)  [unwired: 9 in, 2 out]
                    n302 = call <vilib>:"Simple Error Handler.vi"("error in (no error)"=w247) -> ()  [unwired: 4 in, 5 out]
                  }
                  frame "86 % effective Diameter" {
                    n303 = call "Control 86.vi"() -> ("error out"=w248:errorcluster)  [unwired: 9 in, 2 out]
                    n304 = call <vilib>:"Simple Error Handler.vi"("error in (no error)"=w248) -> ()  [unwired: 4 in, 5 out]
                  }
                }
              }
            }
          }
          event "Display": Value Change {
            n305 = event-data() -> ("NewVal"=w250:T1)  [unwired: 1 in]
            n306 = local read "ok for com"() -> (w251:bool)
            n307 = case shown="False" w251 {
              tunnel: w250 -> [_ w255]
              tunnel: [FALSE ("Visible") w254] -> w249
              frame False {
                n308 = One Button Dialog(message="Not connected to PC-Beamage Software") -> ()  [unwired: 1 in, 1 out]
              }
              frame True {
                n309 = case shown="\"Beam Track Display\"" w255 {
                  tunnel: [FALSE ("Visible") FALSE ("Visible") TRUE ("Visible") FALSE ("Visible")] -> w254
                  frame "2D Display", Default {
                    w256 = FALSE ("Visible")
                    n310 = call "Display 2D.vi"() -> ("error out"=w258:errorcluster)  [unwired: 9 in, 2 out]
                    n311 = call <vilib>:"Simple Error Handler.vi"("error in (no error)"=w258) -> ()  [unwired: 4 in, 5 out]
                    n312 = property on="FWHM On" class="Bool (strict)"("Visible"=w256) -> ()  [unwired: 2 in, 2 out]
                    n313 = property on="Log on" class="Bool (strict)"("Visible"=w256) -> ()  [unwired: 2 in, 2 out]
                    n314 = property on="Gauss on" class="Bool (strict)"("Visible"=w256) -> ()  [unwired: 2 in, 2 out]
                    n315 = property on="1ovre on" class="Bool (strict)"("Visible"=w256) -> ()  [unwired: 2 in, 2 out]
                  }
                  frame "3D Display" {
                    w259 = FALSE ("Visible")
                    n316 = call "Display 3D.vi"() -> ("error out"=w261:errorcluster)  [unwired: 9 in, 2 out]
                    n317 = call <vilib>:"Simple Error Handler.vi"("error in (no error)"=w261) -> ()  [unwired: 4 in, 5 out]
                    n318 = property on="FWHM On" class="Bool (strict)"("Visible"=w259) -> ()  [unwired: 2 in, 2 out]
                    n319 = property on="Log on" class="Bool (strict)"("Visible"=w259) -> ()  [unwired: 2 in, 2 out]
                    n320 = property on="Gauss on" class="Bool (strict)"("Visible"=w259) -> ()  [unwired: 2 in, 2 out]
                    n321 = property on="1ovre on" class="Bool (strict)"("Visible"=w259) -> ()  [unwired: 2 in, 2 out]
                  }
                  frame "XY Display" {
                    w262 = FALSE ("Visible")
                    n322 = call "Display XY.vi"() -> ("error out"=w264:errorcluster)  [unwired: 9 in, 2 out]
                    n323 = call <vilib>:"Simple Error Handler.vi"("error in (no error)"=w264) -> ()  [unwired: 4 in, 5 out]
                    n324 = property on="FWHM On" class="Bool (strict)"("Visible"=w262) -> ()  [unwired: 2 in, 2 out]
                    n325 = property on="Log on" class="Bool (strict)"("Visible"=w262) -> ()  [unwired: 2 in, 2 out]
                    n326 = property on="Gauss on" class="Bool (strict)"("Visible"=w262) -> ()  [unwired: 2 in, 2 out]
                    n327 = property on="1ovre on" class="Bool (strict)"("Visible"=w262) -> ()  [unwired: 2 in, 2 out]
                  }
                  frame "Beam Track Display" {
                    w265 = FALSE ("Visible")
                    n328 = call "Display TRACK.vi"() -> ("error out"=w267:errorcluster)  [unwired: 9 in, 2 out]
                    n329 = call <vilib>:"Simple Error Handler.vi"("error in (no error)"=w267) -> ()  [unwired: 4 in, 5 out]
                    n330 = property on="FWHM On" class="Bool (strict)"("Visible"=w265) -> ()  [unwired: 2 in, 2 out]
                    n331 = property on="Log on" class="Bool (strict)"("Visible"=w265) -> ()  [unwired: 2 in, 2 out]
                    n332 = property on="Gauss on" class="Bool (strict)"("Visible"=w265) -> ()  [unwired: 2 in, 2 out]
                    n333 = property on="1ovre on" class="Bool (strict)"("Visible"=w265) -> ()  [unwired: 2 in, 2 out]
                  }
                }
              }
            }
            n334 = property on="Display" class="Enum (strict)"("Caption.Visible"=w249) -> ()  [unwired: 2 in, 2 out]
            n335 = property on="Log" class="Bool (strict)"("Visible"=w249) -> ()  [unwired: 2 in, 2 out]
            n336 = property on="Gauss" class="Bool (strict)"("Visible"=w249) -> ()  [unwired: 2 in, 2 out]
            n337 = property on="FWHM" class="Bool (strict)"("Visible"=w249) -> ()  [unwired: 2 in, 2 out]
            n338 = property on="1ovre" class="Bool (strict)"("Visible"=w249) -> ()  [unwired: 2 in, 2 out]
          }
          event "Center :": Value Change {
            n339 = event-data() -> ("NewVal"=w268:enum16{"Centroid", "Peak"})  [unwired: 1 in]
            n340 = local read "ok for com"() -> (w269:bool)
            n341 = case shown="False" w269 {
              tunnel: w268 -> [_ w271]
              frame False {
                n342 = One Button Dialog(message="Not connected to PC-Beamage Software") -> ()  [unwired: 1 in, 1 out]
              }
              frame True {
                n343 = case shown="\"Centroid\", Default" w271 {
                  frame "Centroid", Default {
                    n344 = call "Control Centroid.vi"() -> ("error out"=w272:errorcluster)  [unwired: 9 in, 2 out]
                    n345 = call <vilib>:"Simple Error Handler.vi"("error in (no error)"=w272) -> ()  [unwired: 4 in, 5 out]
                  }
                  frame "Peak" {
                    n346 = call "Control Peak.vi"() -> ("error out"=w273:errorcluster)  [unwired: 9 in, 2 out]
                    n347 = call <vilib>:"Simple Error Handler.vi"("error in (no error)"=w273) -> ()  [unwired: 4 in, 5 out]
                  }
                }
              }
            }
          }
          event "Gauss": Value Change {
            n348 = event-data() -> ("NewVal"=w274:bool)  [unwired: 1 in]
            n349 = local read "ok for com"() -> (w275:bool)
            n350 = case shown="False" w275 {
              tunnel: w274 -> [_ w278]
              frame False {
                w276 = FALSE ("verifiy dll")
                n351 = local write "Gauss"(w276) -> ()
                n352 = local write "Gauss on"(w276) -> ()
                n353 = One Button Dialog(message="Not connected to PC-Beamage Software") -> ()  [unwired: 1 in, 1 out]
              }
              frame True {
                n354 = case shown="True" w278 {
                  frame False {
                  }
                  frame True {
                    n355 = local write "Gauss on"(FALSE ("Gauss on")) -> ()
                    n356 = property on="Gauss on" class="Bool (strict)"("Visible"=TRUE) -> ()  [unwired: 2 in, 2 out]
                    n357 = property on="Gauss" class="Bool (strict)"("Visible"=FALSE) -> ()  [unwired: 2 in, 2 out]
                    n358 = call "Activate Gaussian.vi"() -> ()  [unwired: 9 in, 3 out]
                  }
                }
              }
            }
          }
          event "Log": Value Change {
            n359 = event-data() -> ("NewVal"=w282:bool)  [unwired: 1 in]
            n360 = local read "ok for com"() -> (w283:bool)
            n361 = case shown="False" w283 {
              tunnel: w282 -> [_ w286]
              frame False {
                w284 = FALSE ("verifiy dll")
                n362 = local write "Log on"(w284) -> ()
                n363 = local write "Log"(w284) -> ()
                n364 = One Button Dialog(message="Not connected to PC-Beamage Software") -> ()  [unwired: 1 in, 1 out]
              }
              frame True {
                n365 = case shown="True" w286 {
                  frame False {
                  }
                  frame True {
                    n366 = local write "Log on"(FALSE ("Gauss on")) -> ()
                    n367 = property on="Log on" class="Bool (strict)"("Visible"=TRUE) -> ()  [unwired: 2 in, 2 out]
                    n368 = property on="Log" class="Bool (strict)"("Visible"=FALSE) -> ()  [unwired: 2 in, 2 out]
                    n369 = call "Activate LOG.vi"() -> ()  [unwired: 9 in, 3 out]
                  }
                }
              }
            }
          }
          event "FWHM": Value Change {
            n370 = event-data() -> ("NewVal"=w290:bool)  [unwired: 1 in]
            n371 = local read "ok for com"() -> (w291:bool)
            n372 = case shown="False" w291 {
              tunnel: w290 -> [_ w294]
              frame False {
                w292 = FALSE ("verifiy dll")
                n373 = local write "FWHM On"(w292) -> ()
                n374 = local write "FWHM"(w292) -> ()
                n375 = One Button Dialog(message="Not connected to PC-Beamage Software") -> ()  [unwired: 1 in, 1 out]
              }
              frame True {
                n376 = case shown="True" w294 {
                  frame False {
                  }
                  frame True {
                    n377 = local write "FWHM On"(FALSE ("Gauss on")) -> ()
                    n378 = property on="FWHM On" class="Bool (strict)"("Visible"=TRUE) -> ()  [unwired: 2 in, 2 out]
                    n379 = property on="FWHM" class="Bool (strict)"("Visible"=FALSE) -> ()  [unwired: 2 in, 2 out]
                    n380 = call "Activate FWHM.vi"() -> ()  [unwired: 9 in, 3 out]
                  }
                }
              }
            }
          }
          event "1ovre": Value Change {
            n381 = event-data() -> ("NewVal"=w298:bool)  [unwired: 1 in]
            n382 = local read "ok for com"() -> (w299:bool)
            n383 = case shown="False" w299 {
              tunnel: w298 -> [_ w302]
              frame False {
                w300 = FALSE ("verifiy dll")
                n384 = local write "1ovre on"(w300) -> ()
                n385 = local write "1ovre"(w300) -> ()
                n386 = One Button Dialog(message="Not connected to PC-Beamage Software") -> ()  [unwired: 1 in, 1 out]
              }
              frame True {
                n387 = case shown="True" w302 {
                  frame False {
                  }
                  frame True {
                    n388 = local write "1ovre on"(FALSE ("Gauss on")) -> ()
                    n389 = property on="1ovre on" class="Bool (strict)"("Visible"=TRUE) -> ()  [unwired: 2 in, 2 out]
                    n390 = property on="1ovre" class="Bool (strict)"("Visible"=FALSE) -> ()  [unwired: 2 in, 2 out]
                    n391 = call "Activate 1OVRE.vi"() -> ()  [unwired: 9 in, 3 out]
                  }
                }
              }
            }
          }
          event "Gauss on": Value Change {
            n392 = event-data() -> ("NewVal"=w306:bool)  [unwired: 1 in]
            n393 = local read "ok for com"() -> (w307:bool)
            n394 = case shown="True" w307 {
              tunnel: w306 -> [_ w310]
              frame False {
                w308 = FALSE ("verifiy dll")
                n395 = local write "Gauss"(w308) -> ()
                n396 = local write "Gauss on"(w308) -> ()
                n397 = One Button Dialog(message="Not connected to PC-Beamage Software") -> ()  [unwired: 1 in, 1 out]
              }
              frame True {
                n398 = case shown="False" w310 {
                  frame False {
                  }
                  frame True {
                    n399 = local write "Gauss"(FALSE ("Gauss")) -> ()
                    n400 = property on="Gauss" class="Bool (strict)"("Visible"=TRUE) -> ()  [unwired: 2 in, 2 out]
                    n401 = property on="Gauss on" class="Bool (strict)"("Visible"=FALSE) -> ()  [unwired: 2 in, 2 out]
                  }
                }
              }
            }
          }
          event "Log on": Value Change {
            n402 = event-data() -> ("NewVal"=w314:bool)  [unwired: 1 in]
            n403 = local read "ok for com"() -> (w315:bool)
            n404 = case shown="False" w315 {
              tunnel: w314 -> [_ w318]
              frame False {
                w316 = FALSE ("verifiy dll")
                n405 = local write "Log"(w316) -> ()
                n406 = local write "Log on"(w316) -> ()
                n407 = One Button Dialog(message="Not connected to PC-Beamage Software") -> ()  [unwired: 1 in, 1 out]
              }
              frame True {
                n408 = case shown="True" w318 {
                  frame False {
                  }
                  frame True {
                    n409 = local write "Log"(FALSE ("Gauss")) -> ()
                    n410 = property on="Log" class="Bool (strict)"("Visible"=TRUE) -> ()  [unwired: 2 in, 2 out]
                    n411 = property on="Log on" class="Bool (strict)"("Visible"=FALSE) -> ()  [unwired: 2 in, 2 out]
                    n412 = call "Activate LIN.vi"() -> ()  [unwired: 9 in, 3 out]
                  }
                }
              }
            }
          }
          event "FWHM On": Value Change {
            n413 = event-data() -> ("NewVal"=w322:bool)  [unwired: 1 in]
            n414 = local read "ok for com"() -> (w323:bool)
            n415 = case shown="False" w323 {
              tunnel: w322 -> [_ w326]
              frame False {
                w324 = FALSE ("verifiy dll")
                n416 = local write "FWHM On"(w324) -> ()
                n417 = local write "FWHM"(w324) -> ()
                n418 = One Button Dialog(message="Not connected to PC-Beamage Software") -> ()  [unwired: 1 in, 1 out]
              }
              frame True {
                n419 = case shown="True" w326 {
                  frame False {
                  }
                  frame True {
                    n420 = local write "FWHM"(FALSE ("Gauss")) -> ()
                    n421 = property on="FWHM" class="Bool (strict)"("Visible"=TRUE) -> ()  [unwired: 2 in, 2 out]
                    n422 = property on="FWHM On" class="Bool (strict)"("Visible"=FALSE) -> ()  [unwired: 2 in, 2 out]
                  }
                }
              }
            }
          }
          event "1ovre on": Value Change {
            n423 = event-data() -> ("NewVal"=w330:bool)  [unwired: 1 in]
            n424 = local read "ok for com"() -> (w331:bool)
            n425 = case shown="False" w331 {
              tunnel: w330 -> [_ w334]
              frame False {
                w332 = FALSE ("verifiy dll")
                n426 = local write "1ovre on"(w332) -> ()
                n427 = local write "1ovre"(w332) -> ()
                n428 = One Button Dialog(message="Not connected to PC-Beamage Software") -> ()  [unwired: 1 in, 1 out]
              }
              frame True {
                n429 = case shown="True" w334 {
                  frame False {
                  }
                  frame True {
                    n430 = local write "1ovre"(FALSE ("Gauss")) -> ()
                    n431 = property on="1ovre" class="Bool (strict)"("Visible"=TRUE) -> ()  [unwired: 2 in, 2 out]
                    n432 = property on="1ovre on" class="Bool (strict)"("Visible"=FALSE) -> ()  [unwired: 2 in, 2 out]
                  }
                }
              }
            }
          }
          event "Common Measurements": Value Change {
            n433 = event-data() -> ("NewVal"=w338:T2)  [unwired: 1 in]
            n434 = local read "ok for com"() -> (w339:bool)
            n435 = case shown="False" w339 {
              tunnel: w338 -> [_ _]
              frame False {
                n436 = One Button Dialog(message="Not connected to PC-Beamage Software") -> ()  [unwired: 1 in, 1 out]
              }
              frame True {
                n437 = property on="Common Measurements" class="Enum (strict)"() -> ("RingText.Text"=w343:string)  [unwired: 2 in, 2 out]
                n438 = Match Pattern(string=w343, regular expression="Measure") -> (after substring=w341:string)  [unwired: 1 in, 3 out]
                n439 = property on="Common Measurement" class="Str"("Caption.Text"=w341) -> ()  [unwired: 2 in, 2 out]
              }
            }
          }
          event "X Axis Measurements": Value Change {
            n440 = event-data() -> ("NewVal"=w344:T3)  [unwired: 1 in]
            n441 = local read "ok for com"() -> (w345:bool)
            n442 = case shown="False" w345 {
              tunnel: w344 -> [_ w348]
              frame False {
                n443 = One Button Dialog(message="Not connected to PC-Beamage Software") -> ()  [unwired: 1 in, 1 out]
              }
              frame True {
                n444 = property on="X Axis Measurements" class="Enum (strict)"() -> ("RingText.Text"=w351:string)  [unwired: 2 in, 2 out]
                n445 = case shown="\"1/e^2\", Default" w348 {
                  tunnel: [u32 35 ("Text.Font:Size") u32 20 ("Text.Font:Size")] -> w347
                  frame "1/e^2", Default {
                  }
                  frame "Gaussian Equation" {
                  }
                }
                n446 = Format Into String(format string="X Axis %s", w351) -> (resulting string=w349:string)  [unwired: 2 in, 1 out]
                n447 = property on="X Axis Measurement" class="Str"("Caption.Text"=w349) -> ()  [unwired: 2 in, 2 out]
                n448 = property on="X Axis Measurement" class="Str"("Text.FontSize"=w347) -> ()  [unwired: 2 in, 2 out]
              }
            }
          }
          event "Y Axis Measurements": Value Change {
            n449 = event-data() -> ("NewVal"=w354:T3)  [unwired: 1 in]
            n450 = local read "ok for com"() -> (w355:bool)
            n451 = case shown="False" w355 {
              tunnel: w354 -> [_ w358]
              frame False {
                n452 = One Button Dialog(message="Not connected to PC-Beamage Software") -> ()  [unwired: 1 in, 1 out]
              }
              frame True {
                n453 = property on="Y Axis Measurements" class="Enum (strict)"() -> ("RingText.Text"=w361:string)  [unwired: 2 in, 2 out]
                n454 = case shown="\"Gaussian Equation\"" w358 {
                  tunnel: [u32 35 ("Text.Font:Size") u32 20 ("Text.Font:Size")] -> w357
                  frame "1/e^2", Default {
                  }
                  frame "Gaussian Equation" {
                  }
                }
                n455 = Format Into String(format string="Y Axis %s", w361) -> (resulting string=w359:string)  [unwired: 2 in, 1 out]
                n456 = property on="Y Axis Measurement" class="Str"("Caption.Text"=w359) -> ()  [unwired: 2 in, 2 out]
                n457 = property on="Y Axis Measurement" class="Str"("Text.FontSize"=w357) -> ()  [unwired: 2 in, 2 out]
              }
            }
          }
          event "Orientation :": Value Change {
            n458 = event-data() -> ("NewVal"=w364:enum16{"Auto Orient", "0 Degrees", "45 Degress"})  [unwired: 1 in]
            n459 = local read "ok for com"() -> (w365:bool)
            n460 = case shown="False" w365 {
              tunnel: w364 -> [_ w367]
              frame False {
                n461 = One Button Dialog(message="Not connected to PC-Beamage Software") -> ()  [unwired: 1 in, 1 out]
              }
              frame True {
                n462 = case shown="\"Auto Orient\", Default" w367 {
                  frame "Auto Orient", Default {
                    n463 = call "Control Auto.vi"() -> ("error out"=w368:errorcluster)  [unwired: 9 in, 2 out]
                    n464 = call <vilib>:"Simple Error Handler.vi"("error in (no error)"=w368) -> ()  [unwired: 4 in, 5 out]
                  }
                  frame "0 Degrees" {
                    n465 = call "Control Zero.vi"() -> ("error out"=w369:errorcluster)  [unwired: 9 in, 2 out]
                    n466 = call <vilib>:"Simple Error Handler.vi"("error in (no error)"=w369) -> ()  [unwired: 4 in, 5 out]
                  }
                  frame "45 Degress" {
                    n467 = call "Control 45.vi"() -> ("error out"=w370:errorcluster)  [unwired: 9 in, 2 out]
                    n468 = call <vilib>:"Simple Error Handler.vi"("error in (no error)"=w370) -> ()  [unwired: 4 in, 5 out]
                  }
                }
              }
            }
          }
          event "disconnect": Value Change {
            n469 = event-data() -> ()  [unwired: 1 in, 1 out]
            n470 = stacked-sequence {
              frame #0 {
                n471 = local read "Connected"() -> (w371:bool)
                n472 = case shown="False" w371 {
                  frame False {
                    n473 = One Button Dialog(message="Not Connected") -> ()  [unwired: 1 in, 1 out]
                  }
                  frame True {
                    n474 = call "Control Stop Capture.vi"() -> ("error out"=w373:errorcluster)  [unwired: 9 in, 2 out]
                    n475 = call "Disconnect PC Beamage.vi"("error in"=w373) -> ("error out"=w376:errorcluster, "Disconnected"=w375:bool)  [unwired: 9 in]
                    n476 = Not(x=w375) -> (.not. x?=w374:bool)
                    n477 = local write "Connected"(w374) -> ()
                    n478 = call <vilib>:"Simple Error Handler.vi"("error in (no error)"=w376) -> ()  [unwired: 4 in, 5 out]
                  }
                }
              }
              frame #1 {
                w377 = FALSE ("verifiy dll")
                n479 = local write "disconnect"(w377) -> ()
                n480 = local write "Time out"(-1 ("Time out")) -> ()
                n481 = local write "start capture"(w377) -> ()
              }
            }
          }
          event "exit": Value Change {
            n482 = event-data() -> ()  [unwired: 1 in, 1 out]
            n483 = flat-sequence {
              frame #0 {
                n484 = local read "Connected"() -> (w379:bool)
                n485 = case shown="True" w379 {
                  frame False {
                  }
                  frame True {
                    n486 = call "Control Stop Capture.vi"() -> ("error out"=w381:errorcluster)  [unwired: 9 in, 2 out]
                    n487 = call "Disconnect PC Beamage.vi"("error in"=w381) -> ("error out"=w380:errorcluster, "Disconnected"=w383:bool)  [unwired: 9 in]
                    n488 = Not(x=w383) -> (.not. x?=w382:bool)
                    n489 = local write "Connected"(w382) -> ()
                    n490 = call <vilib>:"Simple Error Handler.vi"("error in (no error)"=w380) -> ()  [unwired: 4 in, 5 out]
                  }
                }
              }
              frame #1 {
                w386 = FALSE ("verifiy dll")
                n491 = local write "start capture"(FALSE ("stop capture")) -> ()
                n492 = local write "DLL Present"(w386) -> ()
                n493 = local write "exit"(w386) -> ()
                n494 = property on="start capture" class="Bool (strict)"("Visible"=TRUE) -> ()  [unwired: 2 in, 2 out]
              }
              frame #2 {
                n495 = call "Stay or Go.vi"() -> ()  [unwired: 12 in]
              }
            }
          }
        }
      }
    }
  }
